vi "FrequencyToMilliseconds.vi"(11 "Frequency":dbl) -> (3 "Numeric":i64)   [LabVIEW 2018]
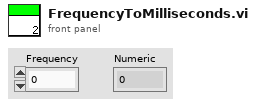
[diagram p1: front panel]
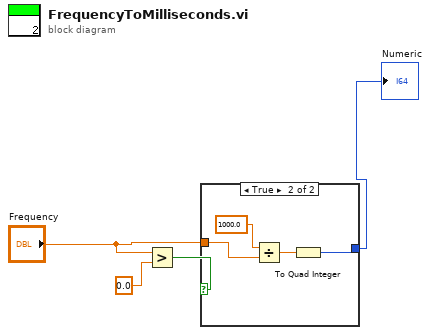
[diagram p0: block diagram]
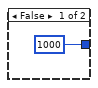
[diagram p2: hidden frame]
diagram:
  n1 = Greater?(x="Frequency", y=0.0) -> (0:w2:bool)
  n2 = case shown="True" w2 {
    tunnel: "Frequency" -> [_ w9]
    tunnel: [i64 1000 w6] -> w4
    frame False {
    }
    frame True {
      n3 = Divide(x=1000.0, y=w9) -> (x/y=w7:dbl)
      n4 = To Quad Integer(1:w7) -> (0:w6:i64)
    }
  }
  "Numeric" <- w4
